vi "Test tag Encode.vi"() -> ()   [LabVIEW 2021]
uses:
  typedef/ISO FD Frame Type.ctl
  CAN_Logic.lvclass
panel:
  out "Echo out":bool
  in  "Echo":bool
  out "ISO FD Type out":T1=enum."CAN 2.0"
  out "Extended ID out":bool
  in  "Extended ID":bool
  in  "ISO FD Type":T1=enum."CAN 2.0"
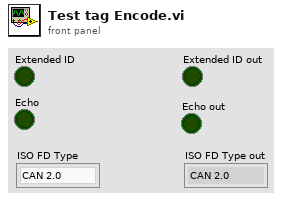
[diagram p1: front panel]
types:
  T1 = typedef "CAN_Logic.lvclass/ISO FD Frame Type.ctl" = enum16{"Not Specified", "CAN 2.0", "FD", "FD+BRS"}
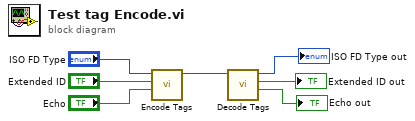
[diagram p0: block diagram]
diagram:
  n1 = call "Encode Tags.vi"("Echo"="Echo", "Extended ID"="Extended ID", "ISO FD Type"="ISO FD Type") -> ("Tags"=w7:u8)  [unwired: 8 in]
  n2 = call "Decode Tags.vi"("Tags in"=w7) -> ("Echo out"=→"Echo out":bool, "Extended ID"=→"Extended ID out":bool, "ISO FD Type"=→"ISO FD Type out":T1)  [unwired: 8 in]
